vi "XIPIN_YCrCb_to_RGB_Color-Space_Converter_7_1.vi"   [LabVIEW 2017]
doc: "The Xilinx YCrCb to RGB Color Space Converter LogiCORE with built-in support for 4 video standards and 3 input ranges. The implementation is a simplified 3x3 constant coefficient matrix multiplier, which uses only 4 multipliers exploiting the inter-relations of color-space conversion coefficients. The module is optimized to take advantage of multiply-add capabilities of DSP slices\n------------------------------------\n<b>Need License</b> : No\n<b>Interface</b> : AXI4 AXI4-Stream"
uses:
  <vilib>/rvi/XilinxIP/XIPIN_XNode/niFpgaXIPIN.xnode
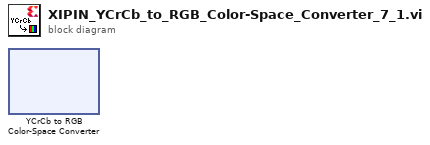
[diagram p0: block diagram]
diagram:
  n1 = xnode ("YCrCb to RGB Color-Space Converter")() -> ()
